vi "Configure Trigger.vi"(0 "VISA resource name":refnum<visa-resource-name>, 1 "Source (0: Immediate)":u16(ring) items=["Immediate", "Timer", "Manual", "Bus", "External"], 2 "Timer Delay (0.001 s)":dbl=0.001, 3 "Count Mode (0: Infinite)":u16(ring) items=["Infinite", "Custom Count"], 4 "Custom Count (1)":i32=1, 5 "error in (no error)":errorcluster, 6 "Auto Delay? (F: Custom)":bool, 8 "Delay (0 s)":dbl, 10 "Init (1: Init Continuous)":i16(ring)=1 items=["Don't Init"=-1, "Init Single"=0, "Init Continuous"=1]) -> (14 "VISA resource name out":refnum<visa-resource-name>, 19 "error out":errorcluster)   [LabVIEW 2015, in "Keithley 2000.lvlib"]
doc: "This VI configures the trigger settings on the instrument."
uses:
  Keithley 2000.lvlib
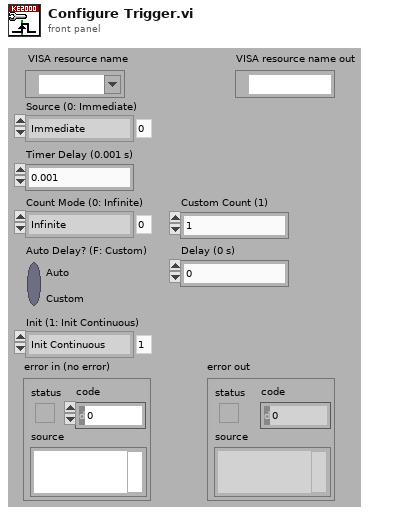
[diagram p1: front panel]
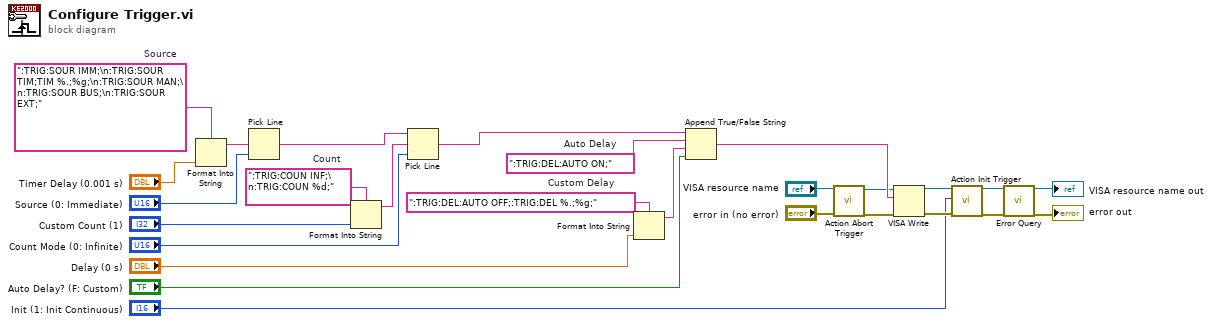
[diagram p0: block diagram]
diagram:
  w18 = ":TRIG:DEL:AUTO ON;"  # Auto Delay
  w21 = ":TRIG:DEL:AUTO OFF;:TRIG:DEL %.;%g;"  # Custom Delay
  w26 = ":TRIG:COUN INF;\n:TRIG:COUN %d;"  # Count
  w15 = ":TRIG:SOUR IMM;\n:TRIG:SOUR TIM;TIM %.;%g;\n:TRIG:SOUR MAN;\n:TRIG:SOUR BUS;\n:TRIG:SOUR EXT;"  # Source
  n1 = Format Into String(format string=w15, "Timer Delay (0.001 s)") -> (resulting string=w13:string)  [unwired: 2 in, 1 out]
  n2 = Pick Line(multi-line string=w13, line index="Source (0: Immediate)") -> (output string=w24:string)  [unwired: 1 in]
  n3 = Format Into String(format string=w26, "Custom Count (1)") -> (resulting string=w25:string)  [unwired: 2 in, 1 out]
  n4 = Pick Line(string ("")=w24, multi-line string=w25, line index="Count Mode (0: Infinite)") -> (output string=w17:string)
  n5 = Format Into String(format string=w21, "Delay (0 s)") -> (resulting string=w19:string)  [unwired: 2 in, 1 out]
  n6 = Append True/False String(1:"Auto Delay? (F: Custom)", 2:w19, 3:w18, 4:w17) -> (0:w12:string)
  n7 = call "Action Abort Trigger.vi"("VISA resource name"="VISA resource name", "error in (no error)"="error in (no error)") -> ("VISA resource name out"=w6:refnum<visa-resource-name>, "error out"=w7:errorcluster)  [unwired: 16 in]
  n8 = VISA Write(VISA resource name=w6, write buffer=w12, error in (no error)=w7) -> (VISA resource name out=w11:refnum<visa-resource-name>, error out=w10:errorcluster)  [unwired: 1 out]
  n9 = call "Action Init Trigger.vi"("VISA resource name"=w11, "Inititiate Mode (1: Init Continuous)"="Init (1: Init Continuous)", "error in (no error)"=w10) -> ("VISA resource name out"=w4:refnum<visa-resource-name>, "error out"=w3:errorcluster)  [unwired: 15 in]
  n10 = call "Error Query.vi"("VISA resource name"=w4, "error in (no error)"=w3) -> ("VISA resource name out"=→"VISA resource name out":refnum<visa-resource-name>, "error out"=→"error out":errorcluster)  [unwired: 14 in, 2 out]
